vi "Built In Object Layout Classes.vi"(8 "error in":errorcluster) -> (0 "error out":errorcluster, 3 "built in object layout classes":refnum<class "Object Layout.lvclass">[](array[class]))   [LabVIEW 2012, in "NI_SE_Front Panel Layout.lvlib"]
uses:
  NI_SE_Front Panel Layout.lvlib
  Object Layout Classes/Object Layout/Object Layout.lvclass
  Object Layout Classes/Control Layout/Control Layout.lvclass
  Object Layout Classes/Text Decoration Layout/Text Decoration Layout.lvclass
  Object Layout Classes/Array Control Layout/Array Control Layout.lvclass
  Object Layout Classes/Cluster Control Layout/Cluster Control Layout.lvclass
  Object Layout Classes/Pane Layout/Pane Layout.lvclass
  Object Layout Classes/Splitter Layout/Splitter Layout.lvclass
  Object Layout Classes/Boolean Control Layout/Boolean Control Layout.lvclass
  Object Layout Classes/Digital Control Layout/Digital Control Layout.lvclass
  Object Layout Classes/NamedNumeric Control Layout/NamedNumeric Control Layout.lvclass
  Object Layout Classes/Listbox Control Layout/Listbox Control Layout.lvclass
  Object Layout Classes/GraphChart Control Layout/GraphChart Control Layout.lvclass
  Object Layout Classes/Tab Control Layout/Tab Control Layout.lvclass
  Object Layout Classes/String Control Layout/String Control Layout.lvclass
  Object Layout Classes/Tree Control Layout/Tree Control Layout.lvclass
  Object Layout Classes/Subpanel Control Layout/Subpanel Control Layout.lvclass
  Object Layout Classes/XControl Layout/XControl Layout.lvclass
  Object Layout Classes/NumericWithScale Control Layout/NumericWithScale Control Layout.lvclass
  Object Layout Classes/Knob Control Layout/Knob Control Layout.lvclass
  Object Layout Classes/Slide Control Layout/Slide Control Layout.lvclass
  Object Layout Classes/Decoration Layout/Decoration Layout.lvclass
  Object Layout Classes/Ring Layout/Ring Layout.lvclass
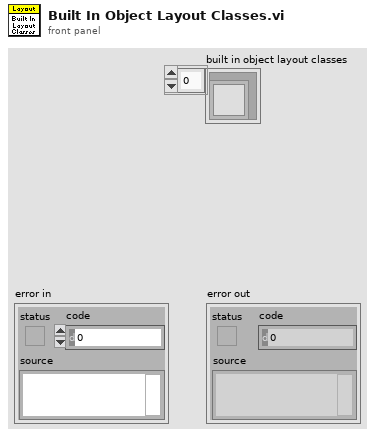
[diagram p1: front panel]
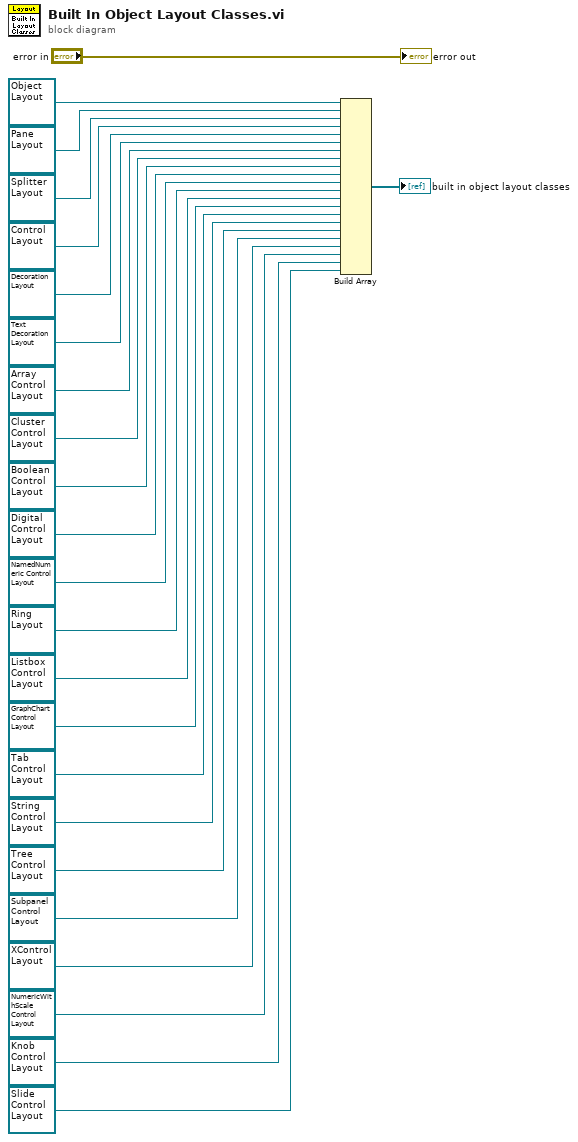
[diagram p0: block diagram]
diagram:
  n1 = Build Array(refnum<class "Object Layout.lvclass"> refnum ("Object Layout.lvclass"), refnum<class "Pane Layout.lvclass"> refnum ("NI_SE_Front Panel Layout.lvlib:NI_SE_Pane Layout.lvclass"), refnum<class "Splitter Layout.lvclass"> refnum ("NI_SE_Front Panel Layout.lvlib:NI_SE_Splitter Layout.lvclass"), refnum<class "Control Layout.lvclass"> refnum ("NI_SE_Front Panel Layout.lvlib:NI_SE_Control Layout.lvclass"), refnum<class "Decoration Layout.lvclass"> refnum ("NI_SE_Front Panel Layout.lvlib:Decoration Layout.lvclass"), refnum<class "Text Decoration Layout.lvclass"> refnum ("NI_SE_Front Panel Layout.lvlib:Text Decoration Layout.lvclass"), refnum<class "Array Control Layout.lvclass"> refnum ("NI_SE_Front Panel Layout.lvlib:NI_SE_Array Control Layout.lvclass"), refnum<class "Cluster Control Layout.lvclass"> refnum ("NI_SE_Front Panel Layout.lvlib:NI_SE_Cluster Control Layout.lvclass"), refnum<class "Boolean Control Layout.lvclass"> refnum ("NI_SE_Front Panel Layout.lvlib:NI_SE_Boolean Control Layout.lvclass"), refnum<class "Digital Control Layout.lvclass"> refnum ("NI_SE_Front Panel Layout.lvlib:NI_SE_Digital Control Layout.lvclass"), refnum<class "NamedNumeric Control Layout.lvclass"> refnum ("NI_SE_Front Panel Layout.lvlib:NI_SE_NamedNumeric Control Layout.lvclass"), refnum<class "Ring Layout.lvclass"> refnum ("NI_SE_Front Panel Layout.lvlib:Ring Layout.lvclass"), refnum<class "Listbox Control Layout.lvclass"> refnum ("NI_SE_Front Panel Layout.lvlib:NI_SE_Listbox Control Layout.lvclass"), refnum<class "GraphChart Control Layout.lvclass"> refnum ("NI_SE_Front Panel Layout.lvlib:NI_SE_GraphChart Control Layout.lvclass"), refnum<class "Tab Control Layout.lvclass"> refnum ("NI_SE_Front Panel Layout.lvlib:NI_SE_Tab Control Layout.lvclass"), refnum<class "String Control Layout.lvclass"> refnum ("NI_SE_Front Panel Layout.lvlib:NI_SE_String Control Layout.lvclass"), refnum<class "Tree Control Layout.lvclass"> refnum ("NI_SE_Front Panel Layout.lvlib:NI_SE_Tree Control Layout.lvclass"), refnum<class "Subpanel Control Layout.lvclass"> refnum ("NI_SE_Front Panel Layout.lvlib:NI_SE_Subpanel Control Layout.lvclass"), refnum<class "XControl Layout.lvclass"> refnum ("NI_SE_Front Panel Layout.lvlib:NI_SE_XControl Layout.lvclass"), refnum<class "NumericWithScale Control Layout.lvclass"> refnum ("NI_SE_Front Panel Layout.lvlib:NumericWithScale Control Layout.lvclass"), refnum<class "Knob Control Layout.lvclass"> refnum ("NI_SE_Front Panel Layout.lvlib:Knob Control Layout.lvclass"), refnum<class "Slide Control Layout.lvclass"> refnum ("NI_SE_Front Panel Layout.lvlib:Slide Control Layout.lvclass")) -> (→"built in object layout classes":refnum<class "Object Layout.lvclass">[])
  "error out" <- "error in"
